vi "EnFlo_Tun_Setup_global.vi"() -> ()   [LabVIEW 2012]
panel:
  out "DB Setup files":string[](array[string])=["EnFlo_Tunnel DB setup.xls", "A_Tunnel DB setup.xls", "D_Tunnel DB setup.xls", "Aero_Tunnel DB setup.xls", "CPP_Tunnel1.xls", "CPP_Tunnel2.xls", "CPP_Tunnel3.xls"]
  in  "CPP Tunnel3 DB array":string[][](array[string])
  in  "CPP Tunnel2 DB array":string[][](array[string])
  in  "CPP Tunnel1 DB array":string[][](array[string])
  in  "Aero Tunnel DB array":string[][](array[string])
  in  "D Tunnel DB array":string[][](array[string])
  in  "A Tunnel DB array":string[][](array[string])
  in  "EnFlo Tun DB array":string[][](array[string])
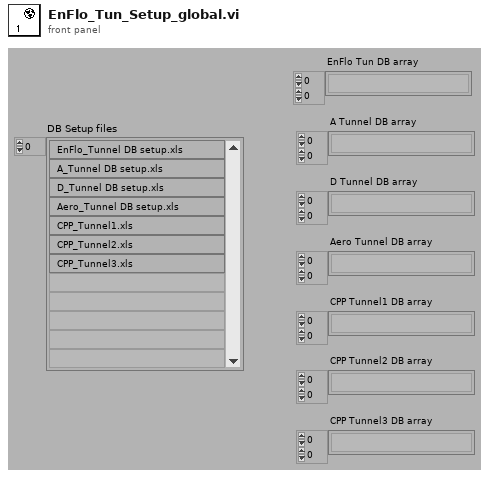
[diagram p1: front panel]
diagram:
